vi "VariablesToString_Scalar.vi"(1 "Terminate?":bool=TRUE, 2 "ValueIn":dbl, 3 "KeyWord":string) -> (0 "StringOut":string)   [LabVIEW 2011]
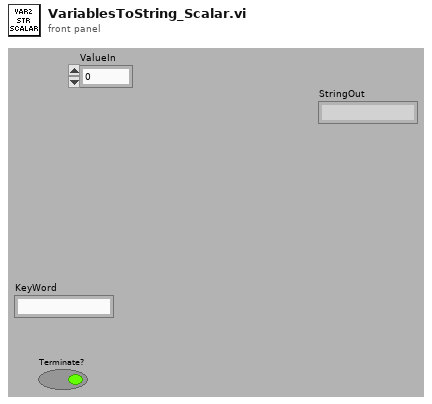
[diagram p1: front panel]
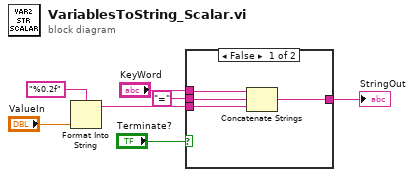
[diagram p0: block diagram]
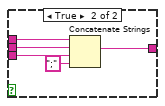
[diagram p2: hidden frame]
diagram:
  n1 = Format Into String(format string="%0.2f", "ValueIn") -> (resulting string=w1:string)  [unwired: 2 in, 1 out]
  n2 = case shown="False" "Terminate?" {
    tunnel: "KeyWord" -> [w11 w16]
    tunnel: "=" ("string") -> [w10 w15]
    tunnel: [w9 w13] -> w4
    tunnel: w1 -> [w8 w12]
    frame False {
      n3 = Concatenate Strings(w11, w10, w8) -> (w9:string)
    }
    frame True {
      n4 = Concatenate Strings(w16, w15, w12, ";" ("string")) -> (w13:string)
    }
  }
  "StringOut" <- w4
